vi "Set Cursor Busy.vi"(8 "error in (no error)":errorcluster) -> (0 "error out":errorcluster)   [LabVIEW 2019, in "Status.lvlib"]
uses:
  Status.lvlib
  Message Queue/State Name.ctl
  Message Queue/Reference Queue.vi
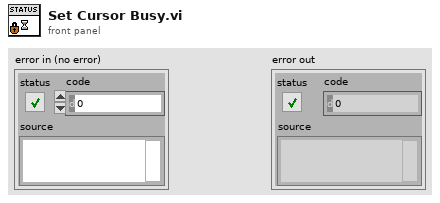
[diagram p1: front panel]
types:
  T1 = typedef "Status.lvlib/State Name.ctl" = enum16{"Initialize", "Update Progress Bar", "Update Status Bar", "Set Cursor Busy", "Unset Cursor Busy", "Error", "Default", "Exit"}
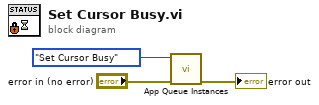
[diagram p0: block diagram]
diagram:
  n1 = call-poly "App Queue Instances.vi"("error in (no error)"="error in (no error)", "Tasks"=State_Name."Set Cursor Busy") -> ("error out"=→"error out":errorcluster)  [unwired: 9 in]
